vi "Open.vi"(8 "error in (no error)":errorcluster, 10 "Address":string, 11 "Instrument.Aerotech in":refnum<class "Instrument.Aerotech.lvclass">) -> (0 "error out":errorcluster, 3 "Instrument.Aerotech out":refnum<class "Instrument.Aerotech.lvclass">)   [LabVIEW 2019, in "Instrument.Aerotech.lvclass"]
uses:
  Instrument.Aerotech.lvclass
  <userlib>/LevyLab/Instrument Framework/Instrument Types/Delay Line/Instrument.DelayLine.lvclass
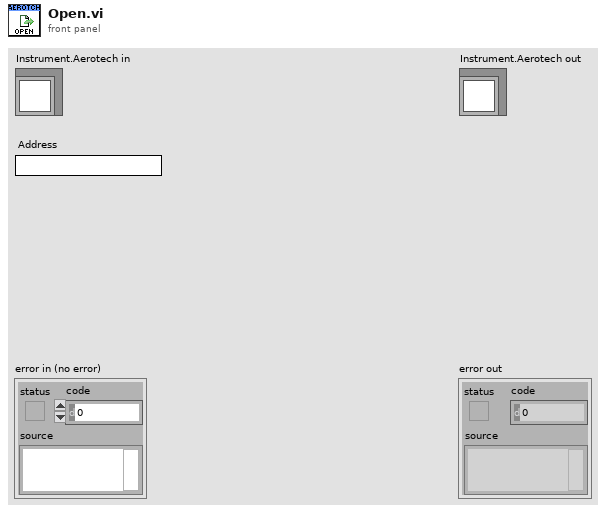
[diagram p1: front panel]
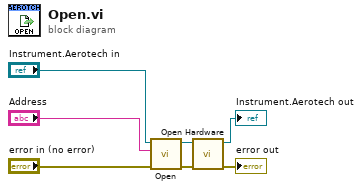
[diagram p0: block diagram]
diagram:
  n1 = call-parent "Open.vi"("error in (no error)"="error in (no error)", "address"="Address", "Instrument in"="Instrument.Aerotech in") -> ("error out"=w3:errorcluster, "Instrument out"=w4:refnum<class "Instrument.Aerotech.lvclass">)  [unwired: 7 in]
  n2 = call-dynamic "Open Hardware.vi"("error in (no error)"=w3, "Instrument.Aerotech in"=w4) -> ("error out"=→"error out":errorcluster, "Instrument.Aerotech out"=→"Instrument.Aerotech out":refnum<class "Instrument.Aerotech.lvclass">)  [unwired: 8 in]
